vi "List Available Measurements.vi"(8 "error in (no error)":errorcluster, 10 "enumerate services request":T1, 11 "multicolumnListbox ref in":refnum<vi>) -> (0 "error out":errorcluster, 1 "create client disabled?":T5(ring), 2 "available measurement details":T2, 3 "multicolumnListbox ref":refnum<vi>, 4 "warning":string, 5 "available measurement names":string[](array[string]))   [LabVIEW 2021, in "MeasurementClient Editor.lvlib"]
uses:
  MeasurementClient Editor.lvlib
  <vilib>/Plug-In SDKs/Clients/Discovery V1/NI Discovery V1 Client.lvlib
  <vilib>/Utility/miscctls.llb/LVRowAndColumnTypeDef.ctl
  <vilib>/gRPC/Generated APIs/ni/measurementlink/discovery/v1/RPC Messages/ni_measurementlink_discovery_v1_ServiceDescriptor_AnnotationsEntry.ctl
  <vilib>/gRPC/Generated APIs/ni/measurementlink/discovery/v1/ni.measurementlink.discovery.v1.api.lvlib
  <vilib>/gRPC/Generated APIs/ni/measurementlink/discovery/v1/RPC Messages/ni_measurementlink_discovery_v1_ServiceDescriptor.ctl
  <vilib>/gRPC/Generated APIs/ni/measurementlink/discovery/v1/RPC Messages/ni_measurementlink_discovery_v1_EnumerateServicesResponse.ctl
  <vilib>/gRPC/Generated APIs/ni/measurementlink/discovery/v1/RPC Messages/ni_measurementlink_discovery_v1_EnumerateServicesRequest.ctl
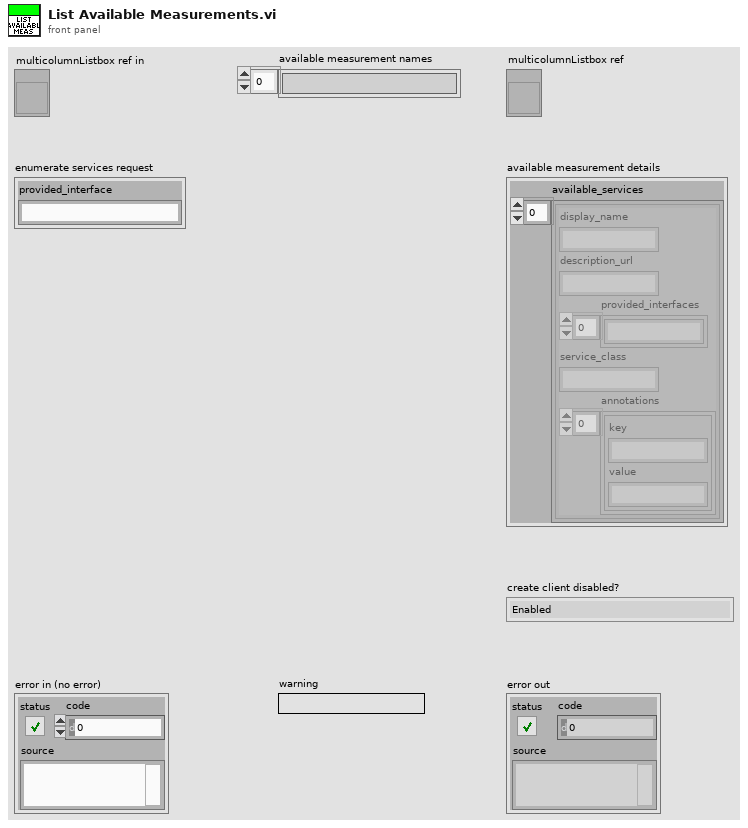
[diagram p1: front panel]
types:
  T1 = typedef "ni.measurementlink.discovery.v1.api.lvlib/ni_measurementlink_discovery_v1_EnumerateServicesRequest.ctl" = cluster{"provided_interface":string}
  T2 = typedef "ni.measurementlink.discovery.v1.api.lvlib/ni_measurementlink_discovery_v1_EnumerateServicesResponse.ctl" = cluster{"available_services":T3[]}
  T3 = typedef "ni.measurementlink.discovery.v1.api.lvlib/ni_measurementlink_discovery_v1_ServiceDescriptor.ctl" = cluster{"display_name":string, "description_url":string, "provided_interfaces":string[], "service_class":string, "annotations":T4[]}
  T4 = typedef "ni.measurementlink.discovery.v1.api.lvlib/ni_measurementlink_discovery_v1_ServiceDescriptor_AnnotationsEntry.ctl" = cluster{"key":string, "value":string}
  T5 = enum8{"Enabled", "Disabled", "Disabled and Grayed Out"}
  T6 = typedef "LVRowAndColumnTypeDef.ctl" = cluster{"Row":i32, "Column":i32}
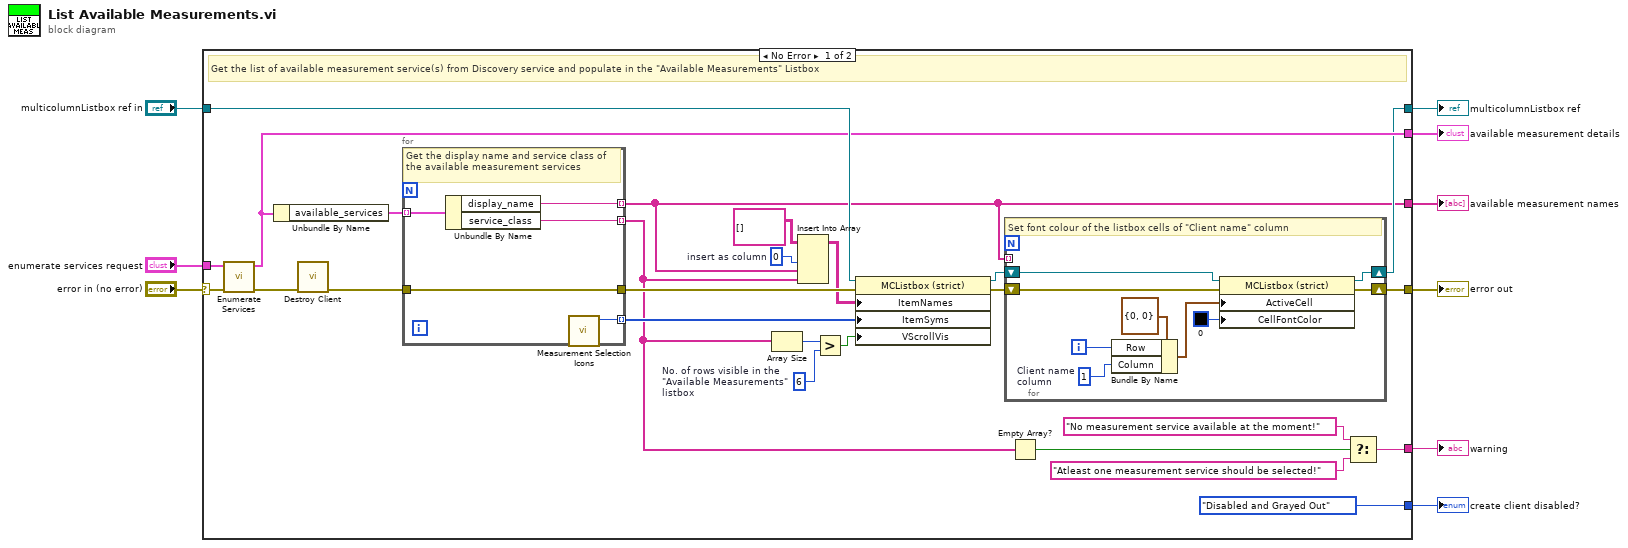
[diagram p0: block diagram]
diagram:
  n1 = case shown="No Error" "error in (no error)" {
    selector: "error in (no error)" -> [w27 w50]
    tunnel: [w20 w50] -> w9
    tunnel: "multicolumnListbox ref in" -> [w34 w51]
    tunnel: [w17 w51] -> w7
    tunnel: [w31 _] -> w6
    tunnel: [w14 _] -> w5
    tunnel: [T5."Disabled and Grayed Out" ("t") _] -> w4
    tunnel: [w26 _] -> w2
    tunnel: "enumerate services request" -> [w25 _]
    frame No Error {
      w12 = 0  # insert as column
      w28 = 6  # No. of rows visible in the "Available Measurements" listbox
      # "Get the list of available measurement service(s) from Discovery service and populate in the \"Available Measurements\" Listbox"
      n2 = call <vilib>:"Enumerate Services.vi"("error in"=w27, "request data"=w25) -> ("error out"=w18:errorcluster, "response data"=w26:T2)  [unwired: 7 in]
      n3 = Unbundle By Name(w26) -> ("available_services"=w11:T3[])
      n4 = call <vilib>:"Destroy Client.vi"("error in"=w18) -> ("error out"=w10:errorcluster)  [unwired: 10 in]
      n5 = for {
        tunnel: w11 -> [w40] mode=indexing
        tunnel: [w38] -> w13 mode=indexing
        tunnel: [w37] -> w33 mode=indexing
        tunnel: [w36] -> w35
        tunnel: [w39] -> w14 mode=indexing
        tunnel: w10 -> [w36]
        # "Get the display name and service class of the available measurement services"
        n6 = Unbundle By Name(w40) -> ("display_name"=w39:string, "service_class"=w38:string)
        n7 = call "Measurement Selection Icons.vi"() -> ("Unchecked"=w37:i32)  [unwired: 10 in, 1 out]
      }
      n8 = Array Size(array=w13) -> (size(s)=w29:i32)
      n9 = Insert Into Array(array=string[][] [], index (col)=w12, new element #1=w14, new element #2=w13) -> (w15:string[][])  [unwired: 1 in]
      n10 = Greater?(x=w29, y=w28) -> (0:w22:bool)
      n11 = property class="MCListbox (strict)"(reference=w34, error in=w35, "ItemNames"=w15, "ItemSyms"=w33, "VScrollVis"=w22) -> (reference out=w19:refnum<vi>, error out=w21:errorcluster)
      n12 = for {
        shift-right: [w48] -> w20
        shift-left: w21 -> [w49]
        tunnel: w14 -> [_] mode=indexing
        shift-right: [w42] -> w17
        shift-left: w19 -> [w47]
        i -> [w44]
        w41 = 1  # Client name column
        # "Set font colour of the listbox cells of \"Client name\" column"
        n13 = Bundle By Name(cluster=T6 {"Row"=0, "Column"=0} ("Active Cell:Active Cell"), "Row"=w44, "Column"=w41) -> (w45:T6)
        n14 = property class="MCListbox (strict)"(reference=w47, error in=w49, "ActiveCell"=w45, "CellFontColor"=u32 0 ("Active Cell:Cell Font:Color")) -> (reference out=w42:refnum<vi>, error out=w48:errorcluster)
      }
      n15 = Empty Array?(array=w13) -> (empty?=w32:bool)
      n16 = Select(t="No measurement service available at the moment!", s=w32, f="Atleast one measurement service should be selected!") -> (s? t:f=w31:string)
    }
    frame Error {
      # "Pass"
    }
  }
  "error out" <- w9
  "multicolumnListbox ref" <- w7
  "create client disabled?" <- w4
  "warning" <- w6
  "available measurement names" <- w5
  "available measurement details" <- w2
